vi "DrawChecked.vi"(8 "error in":errorcluster, 10 "Point":refnum<class "Point.lvclass">, 11 "Color":refnum<class "Color.lvclass">) -> (0 "error out":errorcluster, 3 "Collection out":refnum<class "Collection.lvclass">)   [LabVIEW 2021, in "Menu.lvlib" / "Menu.lvclass"]
uses:
  Menu.lvclass
  Menu.lvclass/Menu.ctl
  Picture2D/src/Line/Line.lvclass
  Picture2D/src/Collection/Collection.lvclass
  Picture2D/src/Point/Point.lvclass
  C:/GitHub/Picture2D/src/Shape/Shape.lvclass
  C:/GitHub/Picture2D/src/Picture2D/Picture2D.lvclass
  C:/GitHub/Picture2D/src/IDrawable/IDrawable.lvclass
  C:/GitHub/Picture2D/src/IMovable/IMovable.lvclass
  C:/GitHub/Picture2D/src/IRotatable/IRotatable.lvclass
  C:/GitHub/Picture2D/src/IScalable/IScalable.lvclass
  C:/GitHub/Picture2D/src/Line/Line.lvclass
  Picture2D/src/Color/Color.lvclass
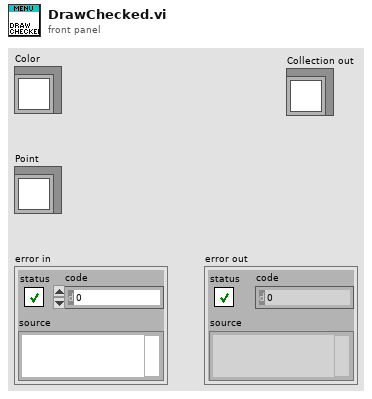
[diagram p1: front panel]
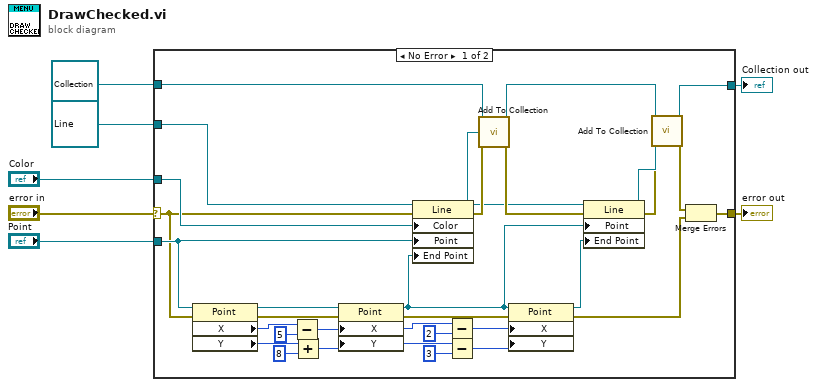
[diagram p0: block diagram]
diagram:
  n1 = case shown="No Error" "error in" {
    selector: "error in" -> [w11 w39]
    tunnel: [w9 w39] -> w7
    tunnel: "Point" -> [w12 _]
    tunnel: "Color" -> [w24 _]
    tunnel: refnum<class "Line.lvclass"> refnum ("Picture2D.lvlib:Line") -> [w37 _]
    tunnel: refnum<class "Collection.lvclass"> refnum ("Picture2D.lvlib:Collection.lvclass") -> [w36 w38]
    tunnel: [w34 w38] -> w1
    frame No Error {
      n2 = property class="Point"(reference=w12, error in=w11) -> (reference out=w13:refnum<class "Point.lvclass">, error out=w15:errorcluster, "X"=w28:i16, "Y"=w26:i16)
      n3 = Subtract(x=w28, y=i16 5) -> (x-y=w10:i16)
      n4 = Add(x=w26, y=i16 8) -> (x+y=w21:i16)
      n5 = property class="Point"(reference=w13, error in=w15, "X"=w10, "Y"=w21) -> (reference out=w17:refnum<class "Point.lvclass">, error out=w14:errorcluster)
      n6 = property class="Line"(reference=w37, error in=w11, "Color"=w24, "Point"=w12, "End Point"=w17) -> (reference out=w16:refnum<class "Line.lvclass">, error out=w32:errorcluster)
      n7 = Subtract(x=w10, y=i16 2) -> (x-y=w23:i16)
      n8 = Subtract(x=w21, y=i16 3) -> (x-y=w20:i16)
      n9 = call-dynamic "Add To Collection.vi"("error in (no error)"=w32, "IDrawable"=w16, "Collection in"=w36) -> ("error out"=w31:errorcluster, "Collection out"=w35:refnum<class "Collection.lvclass">)  [unwired: 7 in]
      n10 = property class="Point"(reference=w17, error in=w14, "X"=w23, "Y"=w20) -> (reference out=w18:refnum<class "Point.lvclass">, error out=w8:errorcluster)
      n11 = property class="Line"(reference=w16, error in=w31, "Point"=w17, "End Point"=w18) -> (reference out=w33:refnum<class "Line.lvclass">, error out=w30:errorcluster)
      n12 = call-dynamic "Add To Collection.vi"("error in (no error)"=w30, "IDrawable"=w33, "Collection in"=w35) -> ("error out"=w29:errorcluster, "Collection out"=w34:refnum<class "Collection.lvclass">)  [unwired: 7 in]
      n13 = Merge Errors(w29, w8) -> (w9:errorcluster)
    }
    frame Error {
    }
  }
  "error out" <- w7
  "Collection out" <- w1
